vi "CreateMessage.vi"(2 "Payload":string, 3 "Operation":u8, 4 "Device":u8=1) -> (1 "Message":string)   [LabVIEW 2021]
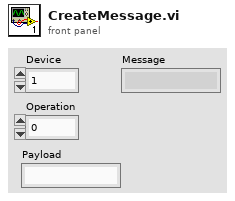
[diagram p1: front panel]
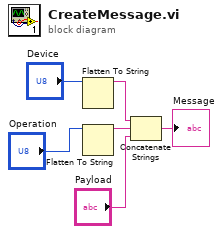
[diagram p0: block diagram]
diagram:
  n1 = Flatten To String(anything="Device") -> (data string=w2:string)  [unwired: 3 in, 2 out]
  n2 = Flatten To String(anything="Operation") -> (data string=w3:string)  [unwired: 3 in, 2 out]
  n3 = Concatenate Strings(w2, w3, "Payload") -> (→"Message":string)
